vi "Initialize with Switch Parameters Core.vi"(8 "error in (no error)":errorcluster, 10 "Switch Parameters in":refnum<class "Abstract Switch Init Parameters.lvclass">=refnum, 11 "SLSC Switch Consumer in":refnum<class "SLSC Switch Consumer.lvclass">=refnum) -> (0 "error out":errorcluster, 3 "SLSC Switch Consumer out":refnum<class "SLSC Switch Consumer.lvclass">)   [LabVIEW 2017, in "NI-SWITCH Messaging.lvlib" / "SLSC Switch Consumer.lvclass"]
uses:
  SLSC Switch Consumer.lvclass
  <vilib>/SLSC_Switch/SLSC Switch.lvlib
  SLSC Switch Init Parameters/SLSC Switch Init Parameters.lvclass
  <vilib>/SLSC_Switch/Initialize with Topology (Simulate).vi
  <vilib>/SLSC_Switch/Initialize with Topology (Override Switches).vi
  Includes/CDMessaging.lvlibp/Switch/Abstract Switch Init Parameters/Abstract Switch Init Parameters.lvclass
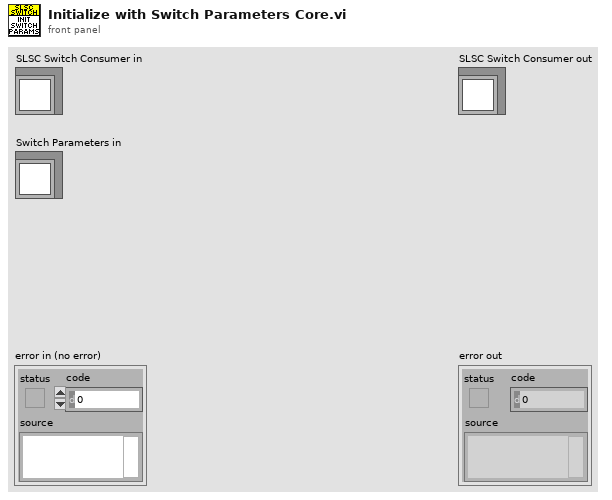
[diagram p1: front panel]
types:
  T1 = typedef "nislscslSession.ctl" = refnum<k20>
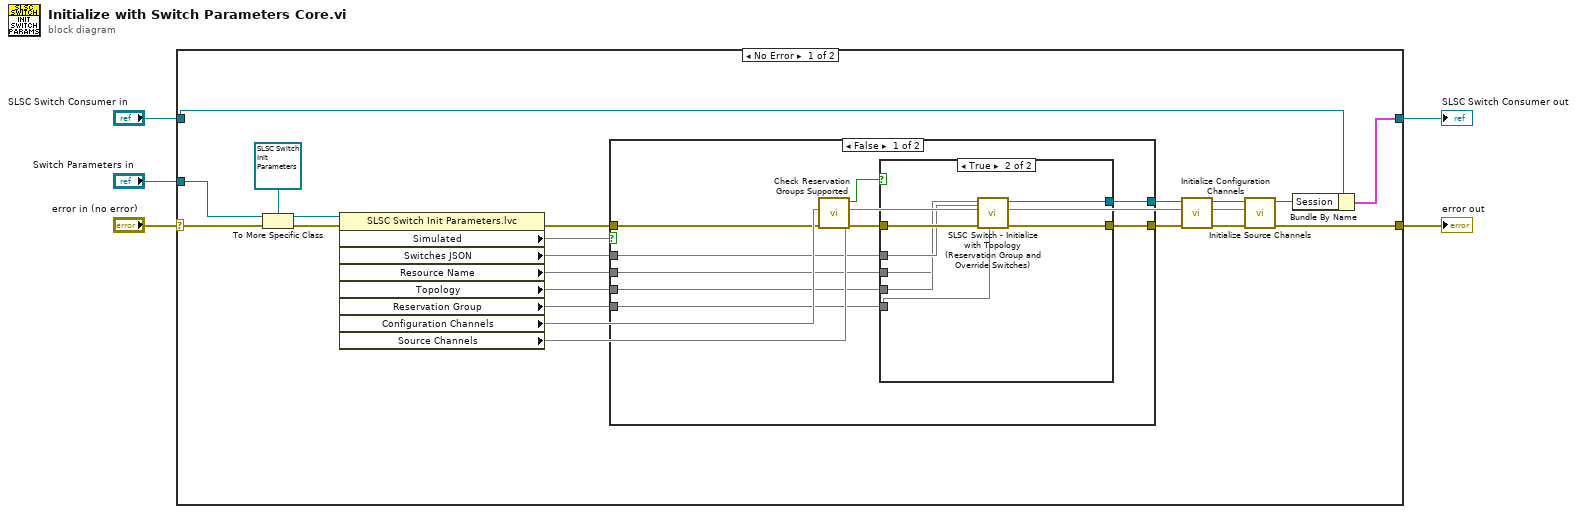
[diagram p0: block diagram]
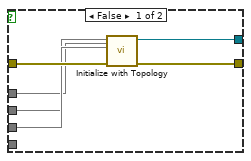
[diagram p2: hidden frame]
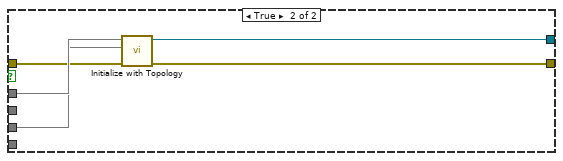
[diagram p3: hidden frame]
diagram:
  n1 = case shown="No Error" "error in (no error)" {
    selector: "error in (no error)" -> [w16 w55]
    tunnel: [w9 w55] -> w4
    tunnel: [w25 w54] -> w1
    tunnel: "SLSC Switch Consumer in" -> [w26 w54]
    tunnel: "Switch Parameters in" -> [w19 _]
    frame No Error {
      n2 = To More Specific Class(target class=refnum<class "SLSC Switch Init Parameters.lvclass"> refnum ("SLSC Switch Messaging.lvlib:SLSC Switch Init Parameters.lvclass"), reference=w19, error in=w16) -> (specific class reference=w17:refnum<class "SLSC Switch Init Parameters.lvclass">, error out=w15:errorcluster)
      n3 = property class="SLSC Switch Init Parameters.lvc"(reference=w17, error in=w15) -> (error out=w23:errorcluster, "Simulated"=w21, "Switches JSON"=w24, "Resource Name"=w22, "Topology"=w20, "Reservation Group"=w7, "Configuration Channels"=w8, "Source Channels"=w6)  [unwired: 1 out]
      n4 = case shown="False" w21 {
        tunnel: w24 -> [w31 w51]
        tunnel: [w34 w53] -> w11
        tunnel: [w35 w52] -> w14
        tunnel: w23 -> [w29 w49]
        tunnel: w22 -> [w32 _]
        tunnel: w20 -> [w33 w50]
        tunnel: w7 -> [w30 _]
        frame False {
          n5 = call "Check Reservation Groups Supported.vi"("error in"=w29) -> ("error out"=w28:errorcluster, "use reservation groups?"=w27:bool)  [unwired: 9 in]
          n6 = case shown="True" w27 {
            tunnel: w28 -> [w41 w48]
            tunnel: [w39 w47] -> w35
            tunnel: [w40 w42] -> w34
            tunnel: w33 -> [w38 w45]
            tunnel: w32 -> [w37 w44]
            tunnel: w31 -> [w36 w46]
            tunnel: w30 -> [_ w43]
            frame False {
              n7 = call-poly <vilib>:"Initialize with Topology.vi"("switches json"=w36, "error in (no error)"=w41, "topology"=w38, "device"=w37) -> ("error out"=w40:errorcluster, "session out"=w39:T1)  [unwired: 6 in]
            }
            frame True {
              n8 = call "SLSC Switch - Initialize with Topology (Reservation Group and Override Switches).vi"("reservation group"=w43, "switches json"=w46, "error in (no error)"=w48, "topology"=w45, "device"=w44) -> ("error out"=w42:errorcluster, "session out"=w47:T1)  [unwired: 5 in]
            }
          }
        }
        frame True {
          n9 = call-poly <vilib>:"Initialize with Topology.vi"("error in (no error)"=w49, "topology"=w50, "switches json"=w51) -> ("error out"=w53:errorcluster, "session out"=w52:T1)  [unwired: 7 in]
        }
      }
      n10 = call "Initialize Configuration Channels.vi"("error in (no error)"=w11, "Configuration Channels"=w8, "Session in"=w14) -> ("error out"=w10:errorcluster, "Session out"=w13:T1)  [unwired: 7 in]
      n11 = call "Initialize Source Channels.vi"("error in (no error)"=w10, "Source Channels"=w6, "Session in"=w13) -> ("error out"=w9:errorcluster, "Session out"=w12:T1)  [unwired: 7 in]
      n12 = Bundle By Name(cluster=w26, "Session"=w12) -> (w25:cluster{})
    }
    frame Error {
    }
  }
  "error out" <- w4
  "SLSC Switch Consumer out" <- w1
